vi "Drop Message Core.vi"(11 "Message in":refnum<class "Message.lvclass">) -> ()   [LabVIEW 2020, in "Actor Framework.lvlib" / "Message.lvclass"]
doc: "<p>(<strong>Filename</strong>: <span class=\"dnl\">Actor Framework.lvlib:Message.lvclass:Drop Message Core.vi</span>)</p>\n<p>Defines what a message does if it is in the message queue when the queue is released. At this point, the actor has shut down, so it will never process the message.</p>\n<p>By default, this method does nothing. A child class may override it to define behavior. National Instruments provides the Reply Msg class to override this method. This class releases its internal queue, which causes any caller of the <a href=\"nihelplauncher://docs/csh?context=lvcore_lvcomm_af_send_and_wait\">Send Message and Wait For Response</a> method to stop waiting and return an error.</p>"
uses:
  Message.lvclass
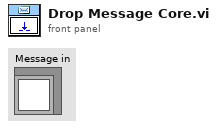
[diagram p1: front panel]
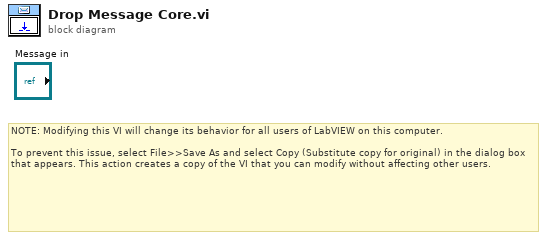
[diagram p0: block diagram]
diagram:
  # "NOTE: Modifying this VI will change its behavior for all users of LabVIEW on this computer.\n\nTo prevent this issue, select File>>Save As and select Copy (Substitute copy for original) in the dialog box that appears. This action creates a copy of the VI that you can modify without affecting other users."
